vi "DigitalIOWrapper.vi"(0 "error in":errorcluster, 2 "Component IDs":string[](array[string]), 3 "True Only (T)":bool=TRUE) -> (1 "error out":errorcluster, 4 "Changed_IO":T1(array[cluster]))   [LabVIEW 2010]
doc: "Fill the Component IDs array with the full names of digital inputs of interest. Returns the name and digital IO state of any input that has changed since last time.\n\nIf True Only is set, then only returns inputs whose value has changed to true (state != 0)"
panel:
  out "changed_io size":i32
  in  "Component":u16(ring) items=["left_lower_cuff", "right_lower_cuff", "left_lower_button", "right_lower_button", "left_upper_button", "right_upper_button", "left_shoulder_button", "right_shoulder_button"]
  in  "EventWrappers":T1(array[cluster])
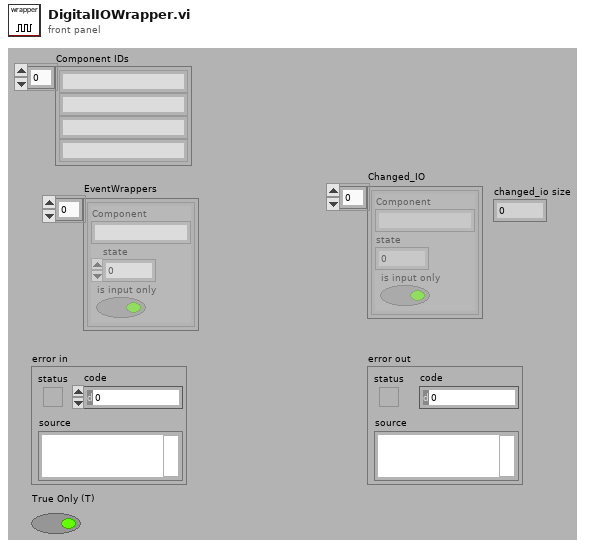
[diagram p1: front panel]
types:
  T1 = cluster{"Component":string, "state":i8, "is input only":bool}[]
  T2 = cluster{"Component":string, "state":i8, "is input only":bool}
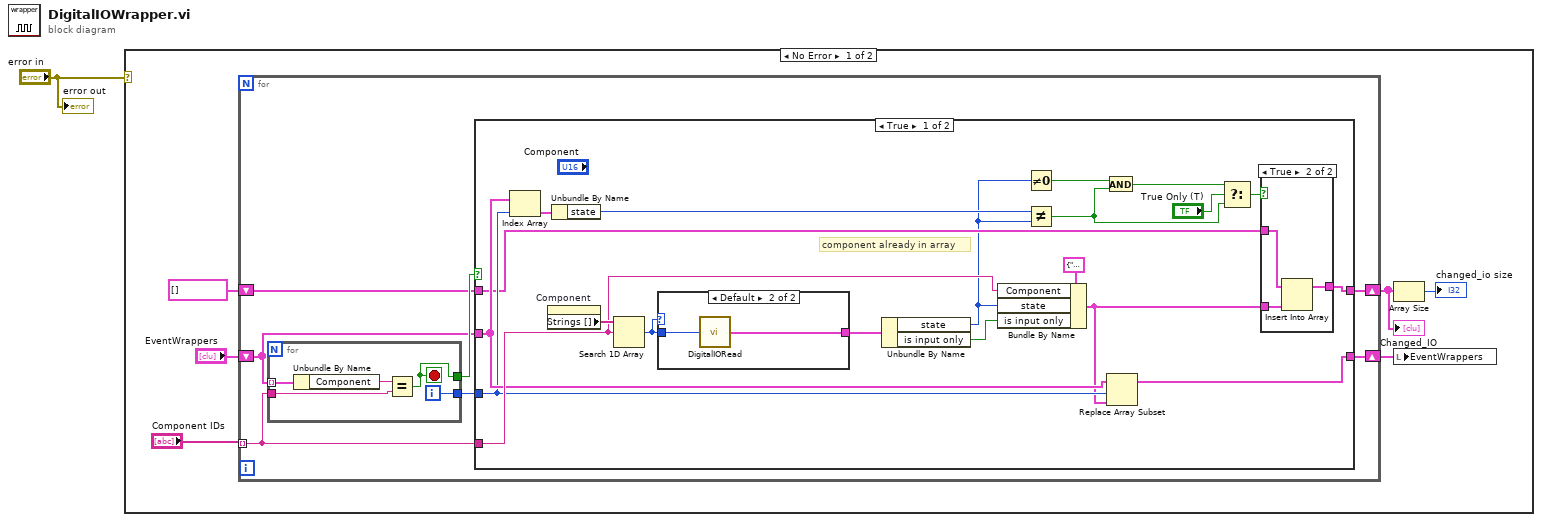
[diagram p0: block diagram]
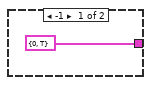
[diagram p2: hidden frame]
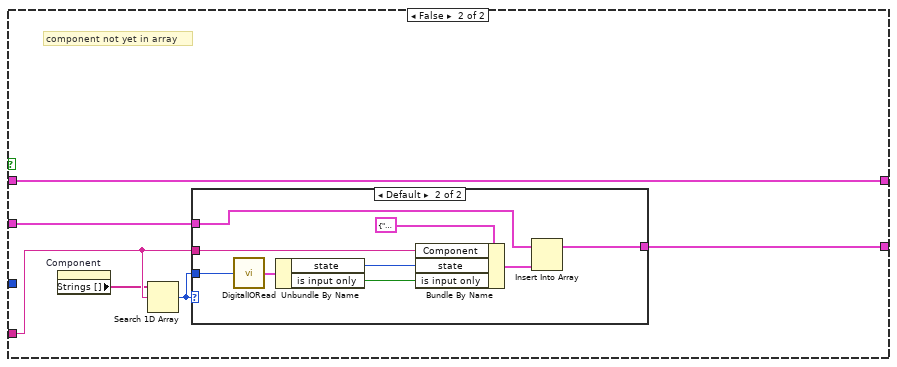
[diagram p4: hidden frame]
diagram:
  n1 = case shown="No Error" "error in" {
    frame No Error {
      n2 = for {
        tunnel: "Component IDs" -> [w8] mode=indexing
        shift-right: [w11] -> w6
        shift-left: "EventWrappers" -> [w12]
        shift-right: [w9] -> w4
        shift-left: T1 [] ("ChangedEvents") -> [w10]
        n3 = for {
          tunnel: w8 -> [w15]
          tunnel: [w16] -> w14
          tunnel: [w19] -> w13
          tunnel: w12 -> [w18] mode=indexing
          i -> [w19]
          stop <- w16 stop-if-true
          n4 = Unbundle By Name(w18) -> ("Component"=w17:string)
          n5 = Equal?(x=w17, y=w15) -> (x = y?=w16:bool)
        }
        n6 = case shown="True" w14 {
          tunnel: w13 -> [w32 _]
          tunnel: w8 -> [w35 w52]
          tunnel: w12 -> [w33 w50]
          tunnel: [w34 w49] -> w11
          tunnel: w10 -> [w29 w48]
          tunnel: [w27 w48] -> w9
          frame True {
            # "component already in array"
            n7 = Index Array(array=w33, index=w32) -> (element=w31:T2)
            n8 = property on="Component" class="Ring (strict)"() -> ("Strings []"=w39:string[])  [unwired: 2 in, 2 out]
            n9 = Unbundle By Name(w31) -> ("state"=w30:i8)
            n10 = Search 1D Array(1D array=w39, element=w35) -> (index of element=w26:i32)  [unwired: 1 in]
            n11 = case shown="Default" w26 {
              tunnel: w26 -> [_ w42]
              tunnel: [cluster{"state":i8, "is input only":bool} {"state"=0, "is input only"=TRUE} ("Digital IO State") w41] -> w37
              frame -1 {
              }
              frame Default {
                n12 = call <userlib>:"DigitalIORead.vi"("Component"=w42) -> ("Digital IO State"=w41:cluster{"state":i8, "is input only":bool})  [unwired: 3 in, 1 out]
              }
            }
            n13 = Unbundle By Name(w37) -> ("state"=w24:i8, "is input only"=w36:bool)
            n14 = Bundle By Name(cluster=T2 {"Component"="", "state"=0, "is input only"=TRUE} ("Digital IO Event Wrapper"), "Component"=w35, "state"=w24, "is input only"=w36) -> (w28:T2)
            n15 = Not Equal To 0?(x=w24) -> (x != 0?=w23:bool)
            n16 = Not Equal?(x=w30, y=w24) -> (x != y?=w21:bool)
            n17 = And(x=w23, y=w21) -> (x .and. y?=w22:bool)
            n18 = Replace Array Subset(array=w33, new element=w28, index=w32) -> (w34:T1)
            n19 = Select(t=w22, s="True Only (T)", f=w21) -> (s? t:f=w20:bool)
            n20 = case shown="True" w20 {
              tunnel: w29 -> [w43 w46]
              tunnel: w28 -> [_ w45]
              tunnel: [w43 w44] -> w27
              frame False {
              }
              frame True {
                n21 = Insert Into Array(array=w46, new element=w45) -> (w44:T1)  [unwired: 1 in]
              }
            }
          }
          frame False {
            # "component not yet in array"
            n22 = property on="Component" class="Ring (strict)"() -> ("Strings []"=w51:string[])  [unwired: 2 in, 2 out]
            n23 = Search 1D Array(1D array=w51, element=w52) -> (index of element=w47:i32)  [unwired: 1 in]
            n24 = case shown="Default" w47 {
              tunnel: w52 -> [_ w59]
              tunnel: w50 -> [w53 w58]
              tunnel: [w53 w56] -> w49
              tunnel: w47 -> [_ w55]
              frame -1 {
              }
              frame Default {
                n25 = call <userlib>:"DigitalIORead.vi"("Component"=w55) -> ("Digital IO State"=w54:cluster{"state":i8, "is input only":bool})  [unwired: 3 in, 1 out]
                n26 = Unbundle By Name(w54) -> ("state"=w61:i8, "is input only"=w60:bool)
                n27 = Bundle By Name(cluster=T2 {"Component"="", "state"=0, "is input only"=TRUE} ("Digital IO Event Wrapper"), "Component"=w59, "state"=w61, "is input only"=w60) -> (w57:T2)
                n28 = Insert Into Array(array=w58, new element=w57) -> (w56:T1)  [unwired: 1 in]
              }
            }
          }
        }
      }
      "Changed_IO" <- w4
      n29 = Array Size(array=w4) -> (size(s)=→"changed_io size":i32)
      n30 = local write "EventWrappers"(w6) -> ()
    }
    frame Error {
    }
  }
  "error out" <- "error in"
